vi "Configure Reference Level.vi"(8 "error in (no error)":errorcluster, 10 "Reference Level [dBm]":dbl, 11 "SA-ESA in":refnum<class "SA-ESA.lvclass">) -> (0 "error out":errorcluster, 3 "SA-ESA out":refnum<class "SA-ESA.lvclass">)   [LabVIEW 2020, in "SA-ESA.lvclass"]
uses:
  SA-ESA.lvclass
  C:/Sandbox/Git_Sandbox/WiSpry Test Framework source code (LV20)/WiSpry Test Framework/Instruments/Instrument.lvclass
  Instrument.lvclass/Instrument.ctl
  Instrument.lvclass
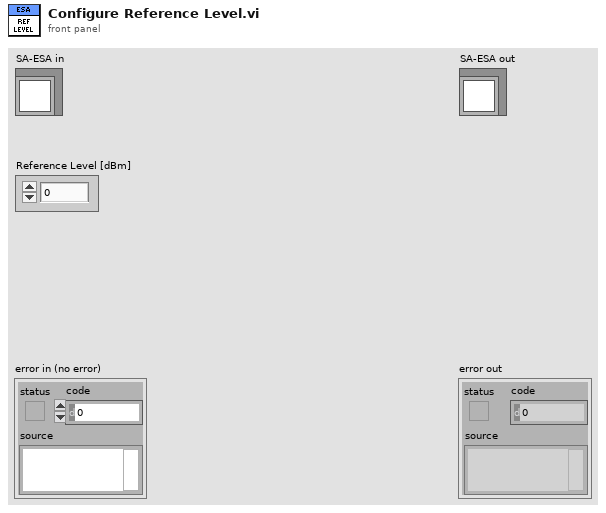
[diagram p1: front panel]
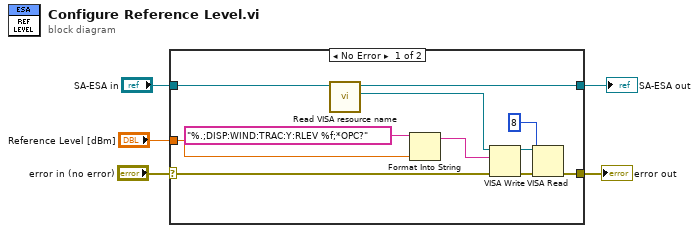
[diagram p0: block diagram]
diagram:
  n1 = case shown="No Error" "error in (no error)" {
    selector: "error in (no error)" -> [w11 w17]
    tunnel: "Reference Level [dBm]" -> [w14 _]
    tunnel: "SA-ESA in" -> [w16 w18]
    tunnel: [w7 w18] -> w2
    tunnel: [w6 w17] -> w1
    frame No Error {
      n2 = call "Read VISA resource name.vi"("Instrument in"=w16) -> ("VISA resource name"=w13:refnum<visa-resource-name>, "Instrument out"=w7:refnum<class "SA-ESA.lvclass">)  [unwired: 9 in]
      n3 = Format Into String(format string="%.;DISP:WIND:TRAC:Y:RLEV %f;*OPC?", w14) -> (resulting string=w12:string)  [unwired: 2 in, 1 out]
      n4 = VISA Write(VISA resource name=w13, write buffer=w12, error in (no error)=w11) -> (VISA resource name out=w9:refnum<visa-resource-name>, error out=w10:errorcluster)  [unwired: 1 out]
      n5 = VISA Read(VISA resource name=w9, byte count=u32 8, error in (no error)=w10) -> (error out=w6:errorcluster)  [unwired: 3 out]
    }
    frame Error {
    }
  }
  "error out" <- w1
  "SA-ESA out" <- w2
